vi "Get VI Name And Description.vi"(8 "Error In":errorcluster, 10 "VI Path":path, 11 "Doc Config":T1) -> (0 "Error Out":errorcluster, 1 "VI Description":string, 2 "VI Name":string, 3 "Doc Config":T1)   [LabVIEW 2011, in "LVH-Toolbox.lvlib" / "LVH-Documentation.lvlib"]
uses:
  LVH-Documentation.lvlib
  Type Defs/Doc Config.ctl
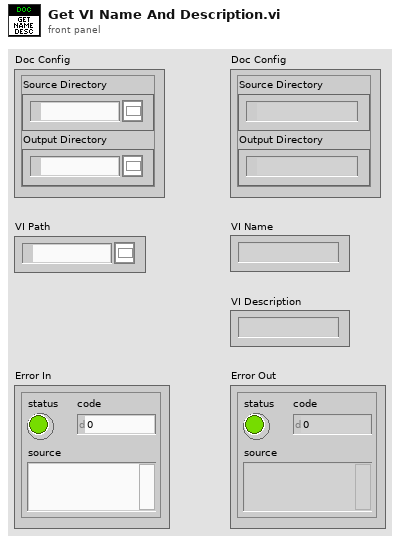
[diagram p1: front panel]
types:
  T1 = typedef "LVH-Toolbox.lvlib/LVH-Documentation.lvlib/Doc Config.ctl" = cluster{"Source Directory":path, "Output Directory":path}
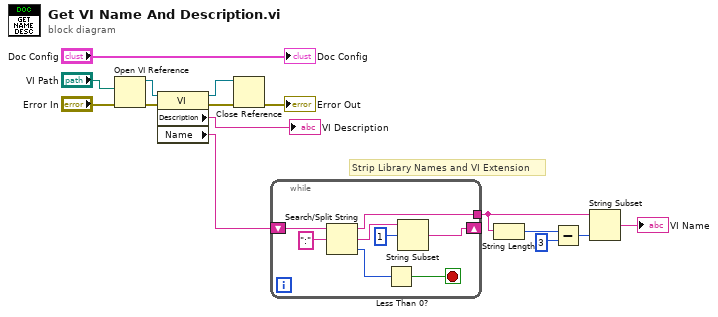
[diagram p0: block diagram]
diagram:
  # "Strip Library Names and VI Extension"
  n1 = Open VI Reference(vi path="VI Path", error in (no error)="Error In") -> (vi reference=w14:refnum<vi>, error out=w12:errorcluster)  [unwired: 4 in]
  n2 = property class="VI"(reference=w14, error in=w12) -> (reference out=w11:refnum<vi>, error out=w10:errorcluster, "Description"=→"VI Description":string, "Name"=w1:string)
  n3 = Close Reference(reference=w11, error in (no error)=w10) -> (error out=→"Error Out":errorcluster)
  n4 = while {
    shift-right: [w20] -> _
    shift-left: w1 -> [w23]
    tunnel: [w16] -> w7
    stop <- w18 stop-if-true
    n5 = Search/Split String(string=w23, search string/char (-)=":") -> (substring before match=w16:string, match + rest of string=w21:string, offset of match=w19:i32)  [unwired: 1 in]
    n6 = Less Than 0?(x=w19) -> (x < 0?=w18:bool)
    n7 = String Subset(string=w21, offset (0)=1) -> (substring=w20:string)  [unwired: 1 in]
  }
  n8 = String Length(string=w7) -> (length=w6:i32)
  n9 = Subtract(x=w6, y=3 ("length (rest)")) -> (x-y=w4:i32)
  n10 = String Subset(string=w7, length (rest)=w4) -> (substring=→"VI Name":string)  [unwired: 1 in]
  "Doc Config" <- "Doc Config"
